vi "MALT160T get one output.vi"() -> ()   [LabVIEW 2018]
uses:
  <instrlib>/AltonTech MALT/AltonTech MALT200817.lvlib
panel:
  in  "Address":i32=3
  in  "Kn":i32=1
  out "Kn Status":bool
  in  "stop":bool
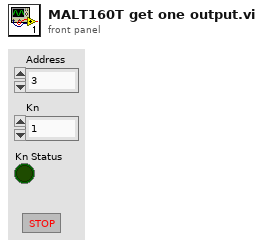
[diagram p1: front panel]
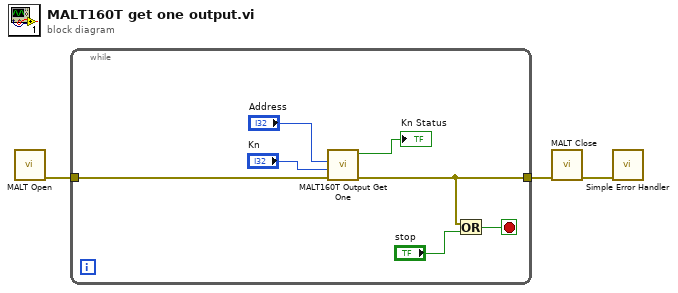
[diagram p0: block diagram]
diagram:
  n1 = call <instrlib>:"MALT Open.vi"() -> ("error out"=w3:errorcluster)  [unwired: 10 in, 1 out]
  n2 = while {
    tunnel: w3 -> [w10]
    tunnel: [w5] -> w2
    stop <- w6 stop-if-true
    n3 = call <instrlib>:"MALT160T Output Get One.vi"("error in"=w10, "Kn"="Kn", "Address"="Address") -> ("error out"=w5:errorcluster, "status"=→"Kn Status":bool)  [unwired: 7 in]
    n4 = Or(x=w5, y="stop") -> (x .or. y?=w6:bool)
  }
  n5 = call <instrlib>:"MALT Close.vi"("error in"=w2) -> ("error out"=w1:errorcluster)  [unwired: 10 in]
  n6 = call <vilib>:"Simple Error Handler.vi"("error in (no error)"=w1) -> ()  [unwired: 4 in, 5 out]
